vi "Open.vi"(8 "error in (no error)":errorcluster, 11 "ENET In":refnum<class "ENET_BS1201.lvclass">) -> (0 "error out":errorcluster, 3 "ENET out":refnum<class "ENET_BS1201.lvclass">)   [LabVIEW 2021, in "BS120x Driver.lvlib" / "ENET_BS1201.lvclass"]
doc: "Open an Ethernet connection to the Battery Simulator 1200 at the specified IP address and ports.\n(c) 2019 Bloomy Controls, Inc. All rights reserved."
uses:
  ENET_BS1201.lvclass
  ENET_BS120x/ENET_BS120x.lvclass
  ENET_BS120x/Async Heartbeat.vi
  C:/Users/Public/Documents/Projects/7100-00109 SW BS1201 LV Driver/trunk/source/ENET_BS120x/ENET_BS120x.lvclass
  C:/Users/Public/Documents/Projects/7100-00109 SW BS1201 LV Driver/trunk/source/BS120x.lvclass
  C:/Users/Public/Documents/Projects/7100-00109 SW BS1201 LV Driver/trunk/source/ENET_BS1201/ENET_BS1201.lvclass
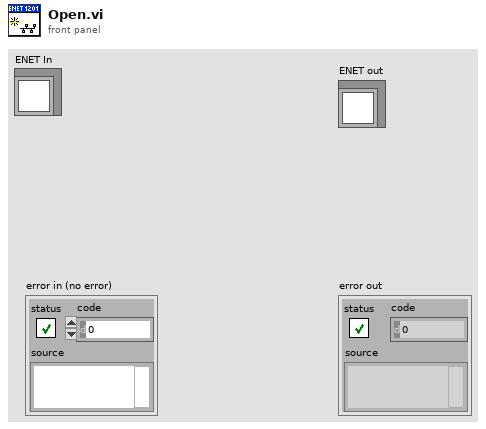
[diagram p1: front panel]
types:
  T1 = typedef "BS120x Driver.lvlib/BS120x.lvclass/Ethernet Settings.ctl" = cluster{"IP Address":string, "TCP (Command) Port":u16, "TCP (Command) Read Interval (ms)":u32, "UDP (Reporting) Port":u16, "UDP (Reporting) Write Interval (ms)":u32, "UDP Data Broadcast Enable":bool}
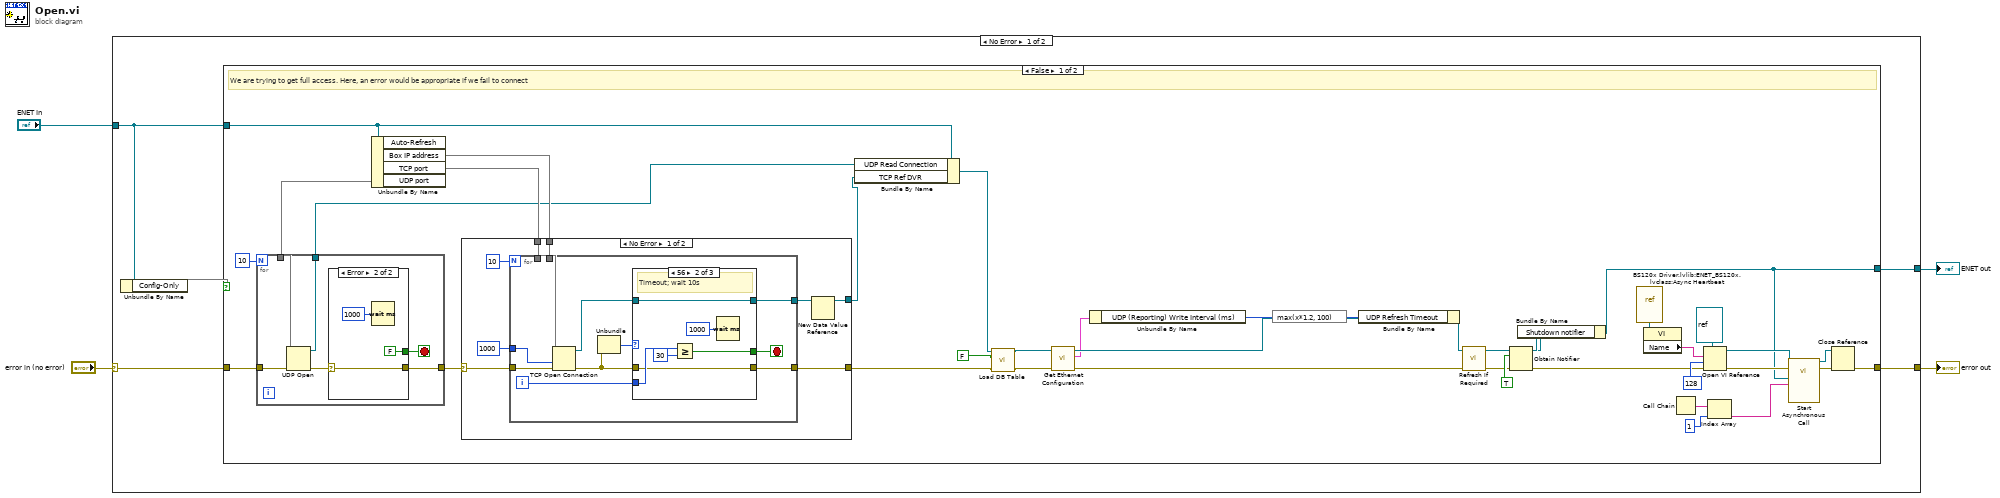
[diagram p0: block diagram]
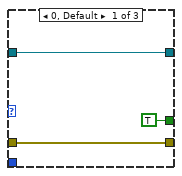
[diagram p2: hidden frame]
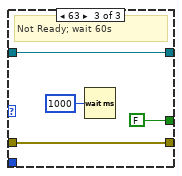
[diagram p3: hidden frame]
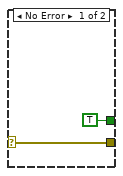
[diagram p5: hidden frame]
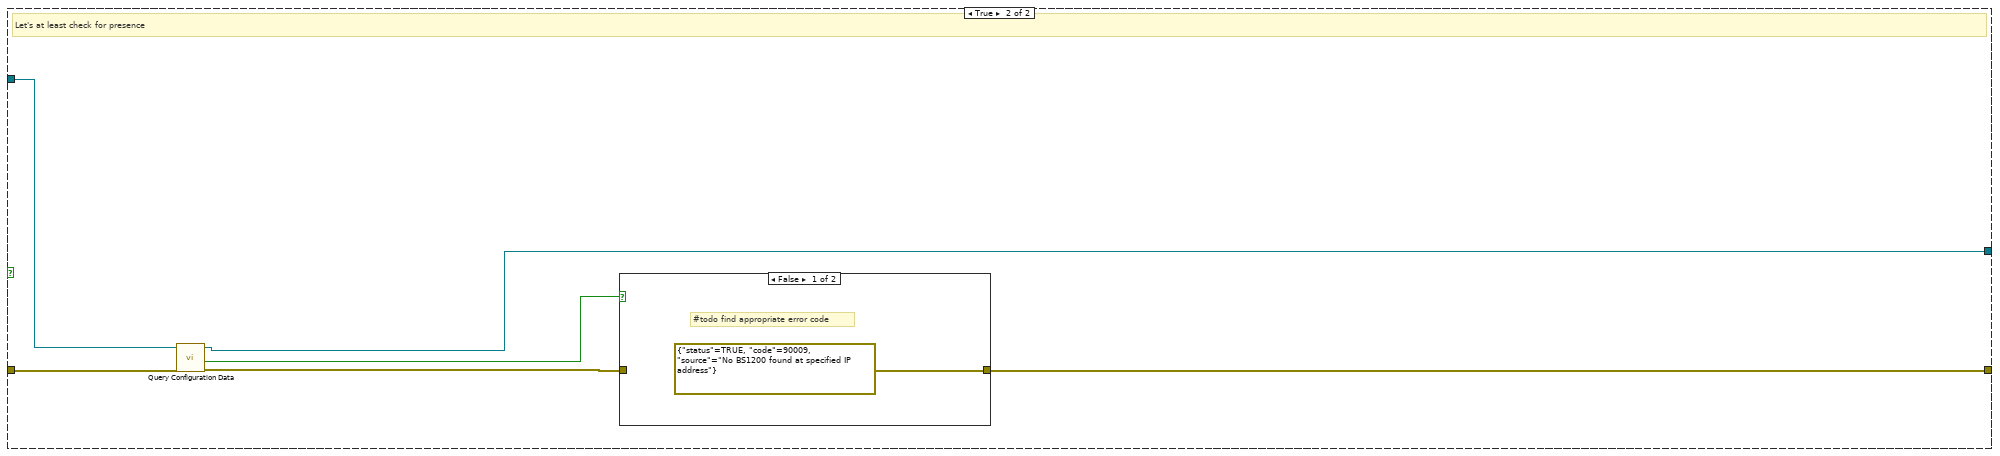
[diagram p6: hidden frame]
diagram:
  n1 = case shown="No Error" "error in (no error)" {
    selector: "error in (no error)" -> [w7 w101]
    tunnel: [w8 w101] -> w3
    tunnel: [w9 w100] -> w2
    tunnel: "ENET In" -> [w6 w100]
    frame No Error {
      n2 = Unbundle By Name(w6) -> ("Config-Only"=w5)
      n3 = case shown="False" w5 {
        tunnel: [w20 w92] -> w9
        tunnel: [w24 w95] -> w8
        tunnel: w6 -> [w17 w93]
        tunnel: w7 -> [w38 w94]
        frame False {
          # "We are trying to get full access. Here, an error would be appropriate if we fail to connect"
          n4 = Unbundle By Name(w17) -> ("Box IP address"=w47, "TCP port"=w46, "UDP port"=w45)  [unwired: 1 out]
          n5 = for {
            N: 10 -> [_]
            tunnel: w45 -> [w85]
            tunnel: [w84] -> w15
            tunnel: w38 -> [w86]
            tunnel: [w82] -> w37
            stop <- w81 stop-if-true
            n6 = UDP Open(8:w86, 11:w85) -> (port=w84:refnum<k16>, 0:w83:errorcluster)  [unwired: 3 in, 1 out]
            n7 = case shown="Error" w83 {
              selector: w83 -> [w88 w90]
              tunnel: [w88 w90] -> w82
              tunnel: [TRUE FALSE] -> w81
              frame No Error {
              }
              frame Error {
                n8 = Wait (ms)(milliseconds to wait=u32 1000) -> ()  [unwired: 1 out]
              }
            }
          }
          n9 = case shown="No Error" w37 {
            selector: w37 -> [w51 w80]
            tunnel: w47 -> [w55 _]
            tunnel: w46 -> [w54 _]
            tunnel: [w50 w80] -> w11
            tunnel: [w48 _] -> w16
            frame No Error {
              n10 = for {
                N: 10 -> [_]
                tunnel: w55 -> [w65]
                tunnel: w54 -> [w64]
                tunnel: 1000 ("timeout ms (25000)") -> [w63]
                tunnel: w51 -> [w66]
                tunnel: [w59] -> w50
                tunnel: [w56] -> w49
                i -> [w62]
                stop <- w61 stop-if-true
                n11 = TCP Open Connection(address=w65, remote port or service name=w64, timeout ms (60000)=w63, error in (no error)=w66) -> (connection ID=w57:refnum<k5>, error out=w58:errorcluster)  [unwired: 1 in]
                n12 = Unbundle(w58) -> ("code"=w60:i32)  [unwired: 2 out]
                n13 = case shown="56" w60 {
                  tunnel: w62 -> [_ w74 _]
                  tunnel: [TRUE w72 FALSE] -> w61
                  tunnel: [w68 w71 w77] -> w59
                  tunnel: w58 -> [w68 w71 w77]
                  tunnel: w57 -> [w67 w70 w76]
                  tunnel: [w67 w70 w76] -> w56
                  frame 0, Default {
                  }
                  frame 56 {
                    # "Timeout; wait 10s"
                    n14 = Greater Or Equal?(x=w74, y=30 ("x")) -> (x >= y?=w72:bool)
                    n15 = Wait (ms)(milliseconds to wait=u32 1000) -> ()  [unwired: 1 out]
                  }
                  frame 63 {
                    # "Not Ready; wait 60s"
                    n16 = Wait (ms)(milliseconds to wait=u32 1000) -> ()  [unwired: 1 out]
                  }
                }
              }
              n17 = New Data Value Reference(data value=w49) -> (data value reference=w48:refnum<data-value>)  [unwired: 1 in, 1 out]
            }
            frame Error {
            }
          }
          n18 = Bundle By Name(cluster=w17, "UDP Read Connection"=w15, "TCP Ref DVR"=w16) -> (w14:refnum<class "ENET_BS1201.lvclass">)
          n19 = call-dynamic "Load DB Table.vi"("error in (no error)"=w11, "Calibration Mode"=FALSE, "ENET in"=w14) -> ("error out"=w10:errorcluster, "ENET out"=w13:refnum<class "ENET_BS1201.lvclass">)  [unwired: 7 in]
          n20 = call-dynamic "Get Ethernet Configuration.vi"("error in (no error)"=w10, "Ethernet in"=w13) -> ("error out"=w43:errorcluster, "Ethernet Settings"=w18:T1, "Ethernet out"=w44:refnum<class "ENET_BS1201.lvclass">)  [unwired: 6 in, 1 out]
          n21 = Unbundle By Name(w18) -> ("UDP (Reporting) Write Interval (ms)"=w41:u32)
          n22 = expression code="max(x*1.2, 100)"(w41) -> (w40:u32)
          n23 = Bundle By Name(cluster=w44, "UDP Refresh Timeout"=w40) -> (w42:refnum<class "ENET_BS1201.lvclass">)
          n24 = call "Refresh If Required.vi"("error in (no error)"=w43, "Ethernet in"=w42) -> ("error out"=w23:errorcluster, "Ethernet out"=w21:refnum<class "ENET_BS1201.lvclass">)  [unwired: 8 in]
          n25 = Obtain Notifier(notification data type=TRUE, error in (no error)=w23) -> (notifier out=w22:refnum<notifier>, error out=w19:errorcluster)  [unwired: 2 in, 1 out]
          n26 = Bundle By Name(cluster=w21, "Shutdown notifier"=w22) -> (w20:refnum<class "ENET_BS1201.lvclass">)
          n27 = vi-ref "BS120x Driver.lvlib:ENET_BS120x.lvclass:Async Heartbeat.vi"() -> (w34:refnum<vi>)
          n28 = property class="VI"(reference=w34) -> ("Name"=w35:string)  [unwired: 1 in, 2 out]
          n29 = Call Chain() -> (call chain=w31:string[])
          n30 = Open VI Reference(type specifier VI Refnum (for type only)=refnum<vi> refnum ("VI Refnum"), vi path=w35, options=128, error in (no error)=w19) -> (vi reference=w28:refnum<vi>, error out=w27:errorcluster)  [unwired: 2 in]
          n31 = Index Array(array=w31, index=1) -> (element=w29:string)
          n32 = call-by-ref "Start Asynchronous Call"(reference=w28, error in=w27, "Main VI"=w29, "Ethernet out"=w20) -> (reference out=w25:refnum<vi>, error out=w26:errorcluster)  [unwired: 10 in]
          n33 = Close Reference(reference=w25, error in (no error)=w26) -> (error out=w24:errorcluster)
        }
        frame True {
          # "Let's at least check for presence"
          n34 = call-dynamic "Query Configuration Data.vi"("error in (no error)"=w94, "Ethernet in"=w93) -> ("error out"=w97:errorcluster, "Received"=w96:bool, "Ethernet out"=w92:refnum<class "ENET_BS1201.lvclass">)  [unwired: 6 in, 1 out]
          n35 = case shown="False" w96 {
            tunnel: w97 -> [_ w99]
            tunnel: [errorcluster {"status"=TRUE, "code"=90009, "source"="No BS1200 found at specified IP address"} ("error constant") w99] -> w95
            frame False {
              # "#todo find appropriate error code"
            }
            frame True {
              # "we're good to go"
            }
          }
        }
      }
    }
    frame Error {
    }
  }
  "error out" <- w3
  "ENET out" <- w2
